vi "Device Selector Changed by user.vi"(10 "Input Cluster":T1, 11 "device":T2) -> (2 "result string":string, 3 "device out":T2)   [LabVIEW 2013]
uses:
  mc device cluster.ctl
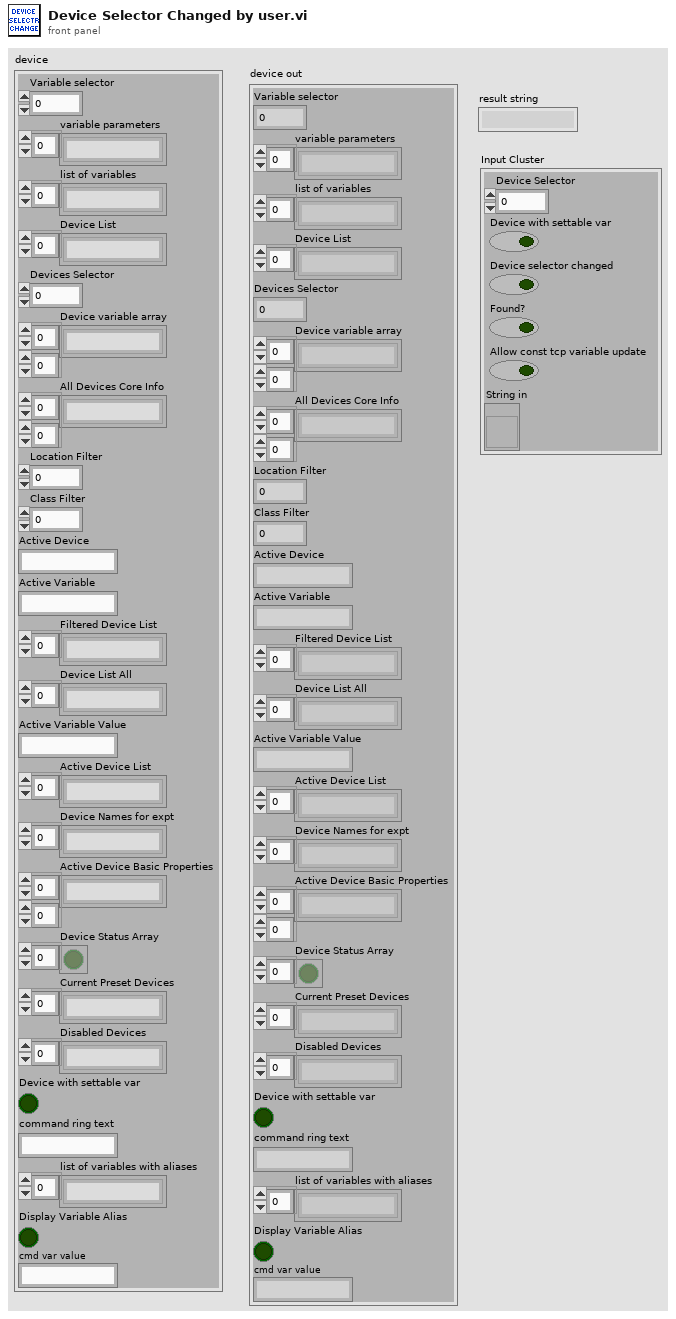
[diagram p1: front panel]
types:
  T1 = cluster{"Device Selector":u16, "Device with settable var":bool, "Device selector changed":bool, "Found?":bool, "Allow const tcp variable update":bool, "String in":refnum<vi>}
  T2 = typedef "mc device cluster.ctl" = cluster{"Variable selector":u16, "variable parameters":string[], "list of variables":string[], "Device List":string[], "Devices Selector":u16, "Device variable array":string[][], "All Devices Core Info":string[][], "Location Filter":u16, "Class Filter":u16, "Active Device":string, "Active Variable":string, "Filtered Device List":string[], "Device List All":string[], "Active Variable Value":string, "Active Device List":string[], "Device Names for expt":string[], "Active Device Basic Properties":string[][], "Device Status Array":bool[], "Current Preset Devices":string[], "Disabled Devices":string[], "Device with settable var":bool, "command ring text":string, "list of variables with aliases":string[], "Display Variable Alias":bool, "cmd var value":string}
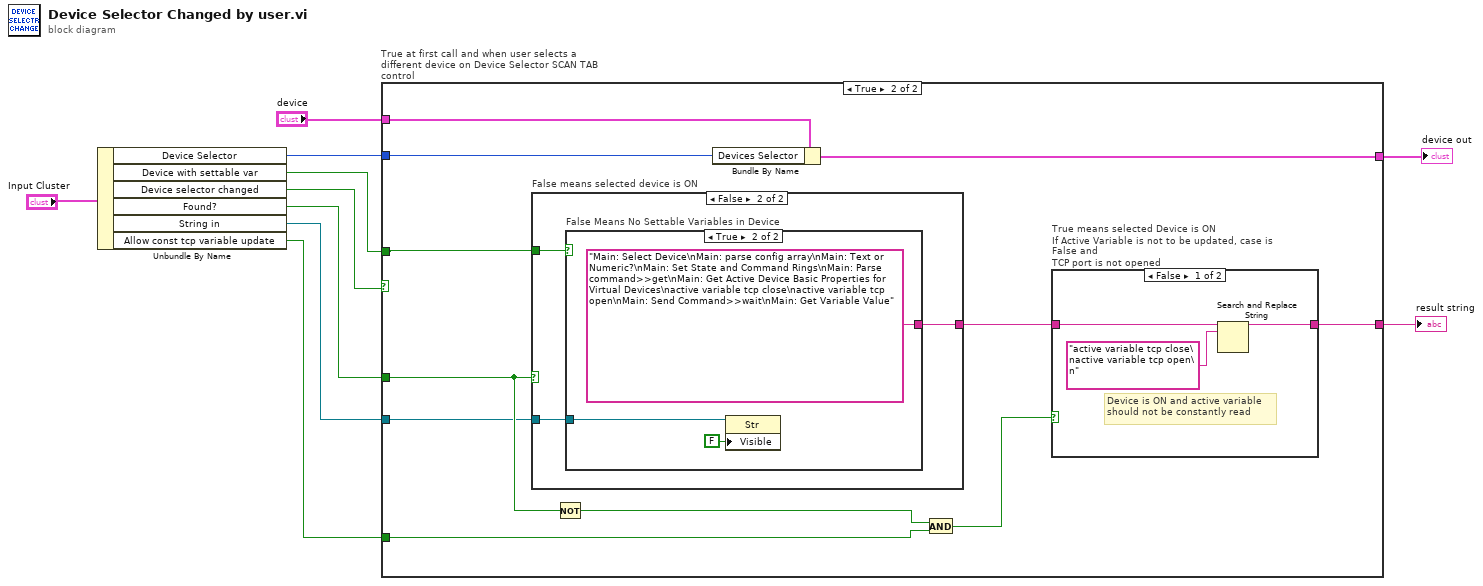
[diagram p0: block diagram]
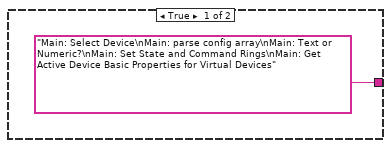
[diagram p3: hidden frame]
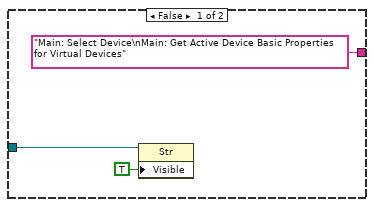
[diagram p4: hidden frame]
diagram:
  n1 = Unbundle By Name("Input Cluster") -> ("Device Selector"=w6:u16, "Device with settable var"=w5:bool, "Device selector changed"=w4:bool, "Found?"=w3:bool, "String in"=w2:refnum<vi>, "Allow const tcp variable update"=w1:bool)
  n2 = case "True at first call and when user selects a different device on Device Selector SCAN TAB control" shown="True" w4 {
    tunnel: [w11 w22] -> w10
    tunnel: [_ w20] -> w8
    tunnel: "device" -> [w11 w19]
    tunnel: w6 -> [_ w18]
    tunnel: w3 -> [_ w17]
    tunnel: w5 -> [_ w14]
    tunnel: w1 -> [_ w13]
    tunnel: w2 -> [_ w12]
    frame False {
    }
    frame True {
      n3 = case "False means selected device is ON" shown="False" w17 {
        tunnel: ["Main: Select Device\nMain: parse config array\nMain: Text or Numeric?\nMain: Set State and Command Rings\nMain: Get Active Device Basic Properties for Virtual Devices" w26] -> w21
        tunnel: w14 -> [_ w25]
        tunnel: w12 -> [_ w24]
        frame True {
        }
        frame False {
          n4 = case "False Means No Settable Variables in Device" shown="True" w25 {
            tunnel: ["Main: Select Device\nMain: Get Active Device Basic Properties for Virtual Devices" "Main: Select Device\nMain: parse config array\nMain: Text or Numeric?\nMain: Set State and Command Rings\nMain: Parse command>>get\nMain: Get Active Device Basic Properties for Virtual Devices\nactive variable tcp close\nactive variable tcp open\nMain: Send Command>>wait\nMain: Get Variable Value"] -> w26
            tunnel: w24 -> [w27 w30]
            frame False {
              n5 = property on="Property Node" class="Str"(reference=w27, "Visible"=TRUE) -> ()  [unwired: 1 in, 2 out]
            }
            frame True {
              n6 = property on="Property Node" class="Str"(reference=w30, "Visible"=FALSE) -> ()  [unwired: 1 in, 2 out]
            }
          }
        }
      }
      n7 = Not(x=w17) -> (.not. x?=w15:bool)
      n8 = Bundle By Name(cluster=w19, "Devices Selector"=w18) -> (w22:T2)
      n9 = And(x=w15, y=w13) -> (x .and. y?=w16:bool)
      n10 = case "True means selected Device is ON\nIf Active Variable is not to be updated, case is False and \nTCP port is not opened" shown="False" w16 {
        tunnel: w21 -> [w34 w36]
        tunnel: [w33 w36] -> w20
        frame False {
          # "Device is ON and active variable\nshould not be constantly read"
          n11 = Search and Replace String(input string=w34, search string="active variable tcp close\nactive variable tcp open\n" ("substring (\"\")")) -> (result string=w33:string)  [unwired: 6 in, 3 out]
        }
        frame True {
          # "Device is ON \nand active variable is to\nbe constantly read"
        }
      }
    }
  }
  "device out" <- w10
  "result string" <- w8
